vi "Viterbi Algorithm.vi"(10 "Observed Sequence":i32[](array[numeric]), 11 "HMM Cluster":T1) -> (2 "Partial Probalility":dbl[][](array[numeric]), 3 "Viterbi Path":i32[](array[numeric]))   [LabVIEW 2014, in "HMM.lvlib"]
uses:
  HMM.lvlib
  Control/HMM Cluster.ctl
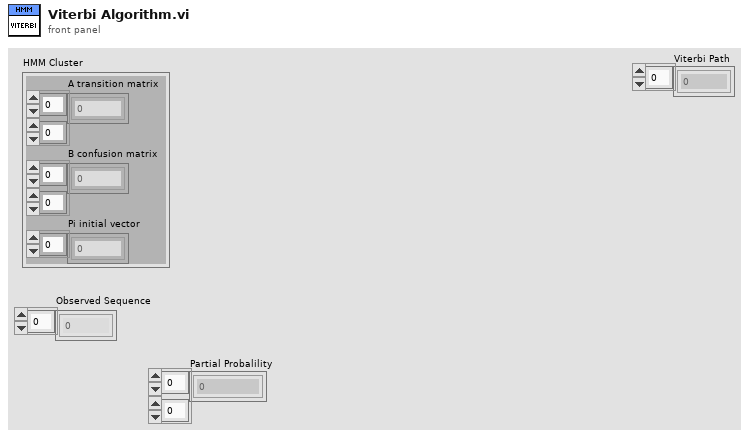
[diagram p1: front panel]
types:
  T1 = typedef "HMM.lvlib/HMM Cluster.ctl" = cluster{"A transition matrix":dbl[][], "B confusion matrix":dbl[][], "Pi initial vector":dbl[]}
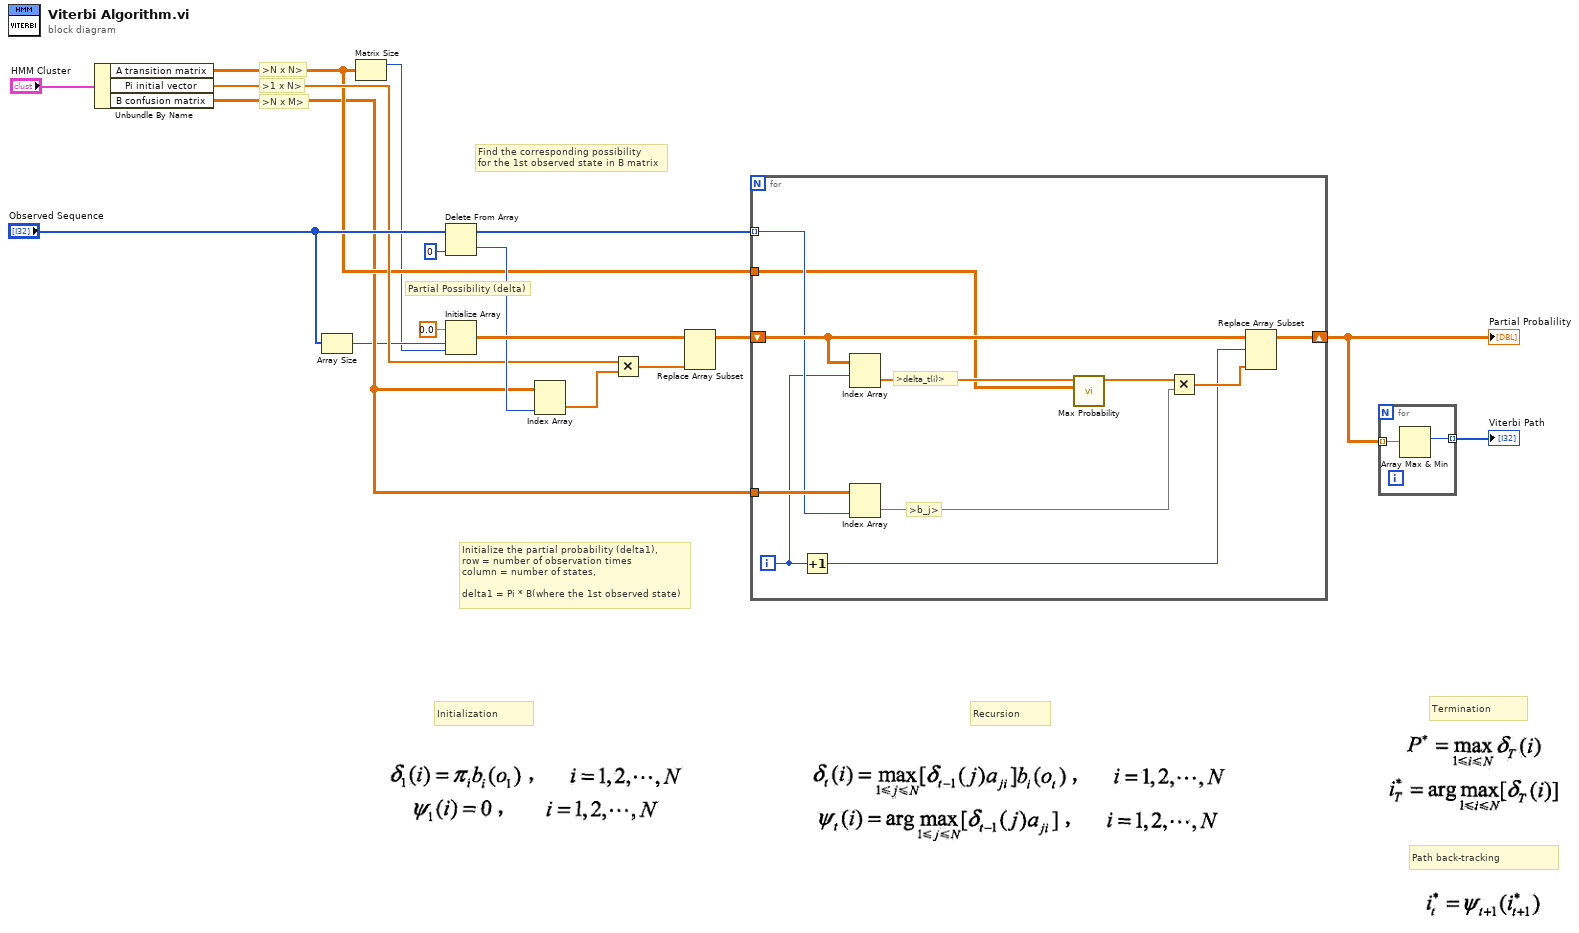
[diagram p0: block diagram]
diagram:
  # "Path back-tracking"
  # "Termination"
  # "Recursion"
  # "Initialization"
  # ">N x M>"
  # ">1 x N>"
  # ">N x N>"
  # "Partial Possibility (delta)"
  # "Find the corresponding possibility\nfor the 1st observed state in B matrix"
  # "Initialize the partial probability (delta1),\nrow = number of observation times\ncolumn = number of states,\n\ndelta1 = Pi * B(where the 1st observed state)"
  n1 = Unbundle By Name("HMM Cluster") -> ("A transition matrix"=w6:dbl[][], "Pi initial vector"=w7:dbl[], "B confusion matrix"=w5:dbl[][])
  n2 = Array Size(array="Observed Sequence") -> (size(s)=w4:i32)
  n3 = Matrix Size(0:w6) -> (1:w1:i32)  [unwired: 1 out]
  n4 = Delete From Array(array="Observed Sequence", index=0) -> (deleted portion=w8:i32, array with subset deleted=w10:i32[])  [unwired: 1 in]
  n5 = Initialize Array(0.0 ("element"), w4, w1) -> (w15:dbl[][])
  n6 = Index Array(array=w5, index (col)=w8) -> (element=w12:dbl[])  [unwired: 1 in]
  n7 = Multiply(x=w7, y=w12) -> (x*y=w11:dbl[])
  n8 = Replace Array Subset(array=w15, new element=w11) -> (w14:dbl[][])  [unwired: 2 in]
  n9 = for {
    tunnel: w10 -> [w25] mode=indexing
    shift-right: [w28] -> w3
    shift-left: w14 -> [w27]
    tunnel: w6 -> [w20]
    tunnel: w5 -> [w26]
    i -> [w22]
    # ">delta_t(i)>"
    # ">b_j>"
    n10 = Increment(x=w22) -> (x+1=w18:i32)
    n11 = Index Array(array=w27, index (row)=w22) -> (element=w21:dbl[])  [unwired: 1 in]
    n12 = Index Array(array=w26, index (col)=w25) -> (element=w24:dbl[])  [unwired: 1 in]
    n13 = call "Max Probability.vi"("A"=w20, "theta_(t-1)"=w21) -> ("Max Probability"=w19:dbl[])  [unwired: 9 in]
    n14 = Multiply(x=w19, y=w24) -> (x*y=w23:dbl[])
    n15 = Replace Array Subset(array=w27, new element=w23, index (row)=w18) -> (w28:dbl[][])  [unwired: 1 in]
  }
  "Partial Probalility" <- w3
  n16 = for {
    tunnel: w3 -> [w30] mode=indexing
    tunnel: [w29] -> w2 mode=indexing
    n17 = Array Max & Min(array=w30) -> (max index (indices)=w29:i32)  [unwired: 3 out]
  }
  "Viterbi Path" <- w2
